vi "Write isObsolete.vi"(8 "error in (no error)":errorcluster, 10 "isObsolete":bool, 11 "_ISerializable in":refnum<class "_ISerializable.lvclass">) -> (0 "error out":errorcluster, 3 "_ISerializable out":refnum<class "_ISerializable.lvclass">)   [LabVIEW 2018, in "_ISerializable.lvclass"]
uses:
  _ISerializable.lvclass
  _ISerializable.lvclass/_ISerializable.ctl
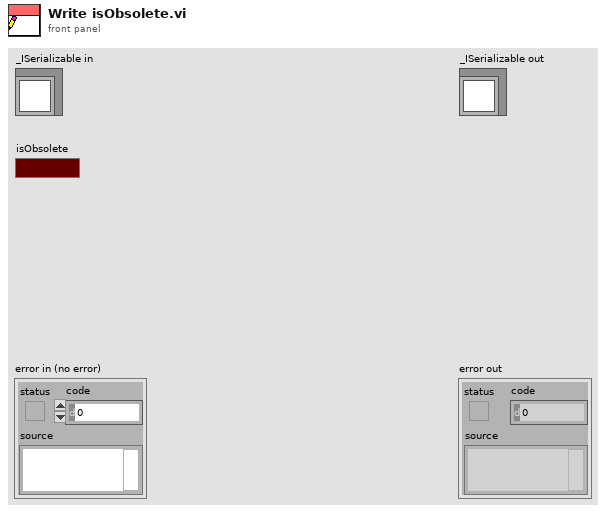
[diagram p1: front panel]
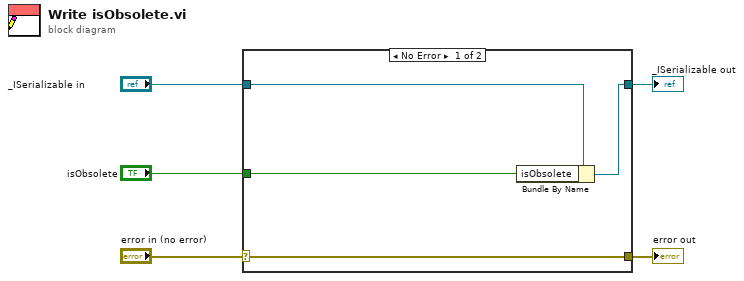
[diagram p0: block diagram]
diagram:
  n1 = case shown="No Error" "error in (no error)" {
    selector: "error in (no error)" -> [w9 w10]
    tunnel: [w9 w10] -> w4
    tunnel: [w7 w11] -> w2
    tunnel: "_ISerializable in" -> [w8 w11]
    tunnel: "isObsolete" -> [w6 _]
    frame No Error {
      n2 = Bundle By Name(cluster=w8, "isObsolete"=w6) -> (w7:refnum<class "_ISerializable.lvclass">)
    }
    frame Error {
    }
  }
  "error out" <- w4
  "_ISerializable out" <- w2
